vi "TCP Chat Window Launcher.vi"() -> ()   [LabVIEW 2020]
uses:
  <vilib>/NI/Actors/Network Endpoint Actors/Protocols/TCP Strategy/TCP Stream Initiator/TCP Stream Initiator.lvclass
  <vilib>/NI/Actors/Network Endpoint Actors/Protocols/TCP Strategy/TCP Stream Listener/TCP Stream Listener.lvclass
  <vilib>/NI/Actors/Network Endpoint Actors/Protocols/TCP Strategy/TCP Stream/TCP Stream.lvclass
  Chat Window/Chat Window.lvclass
  <vilib>/ActorFramework/Actor/Actor.lvclass
  C:/Program Files (x86)/National Instruments/LabVIEW 2020/vi.lib/ActorFramework/Actor/Actor.lvclass
  G:/Utilisateurs/hugofroylan.aragon/Documents/LabVIEW-Projects/Nested Endpoint Actors/Chat Window/Chat Window/Chat Window.lvclass
  C:/Program Files (x86)/National Instruments/LabVIEW 2020/vi.lib/NI/Actors/Network Endpoint Actors/Nested Endpoint Caller/Nested Endpoint Caller/Nested Endpoint Caller.lvclass
  Nested Endpoint Actors/Serializer/Serializable Flattener/Serializable Flattener.lvclass
  G:/Utilisateurs/hugofroylan.aragon/Documents/Nested Endpoint Actors Optimized/Abstract Classes/Message Flattener/Message Flattener.lvclass
  G:/Utilisateurs/hugofroylan.aragon/Documents/LabVIEW-Projects/Nested Endpoint Actors Optimized/Serializer/Serializable Flattener/Serializable Flattener.lvclass
  C:/Program Files (x86)/National Instruments/LabVIEW 2020/vi.lib/NI/Actors/Network Endpoint Actors/Protocols/TCP Strategy/TCP Stream/TCP Stream.lvclass
  G:/Utilisateurs/hugofroylan.aragon/Documents/Nested Endpoint Actors Optimized/Abstract Classes/Message Stream/Message Stream.lvclass
  C:/Program Files (x86)/National Instruments/LabVIEW 2020/vi.lib/NI/Actors/Network Endpoint Actors/Protocols/TCP Strategy/TCP Stream Listener/TCP Stream Listener.lvclass
  C:/Program Files (x86)/National Instruments/LabVIEW 2020/vi.lib/NI/Actors/Network Endpoint Actors/Protocols/TCP Strategy/TCP Stream Initiator/TCP Stream Initiator.lvclass
panel:
  out "error out":errorcluster
  in  "local port":u16=2001
  in  "Remote Port":u16=2001
  in  "Remote Address":string="127.0.0.1"
  # "This VI launches two instances of a chat window actor.  The two chat windows launch nested endpoints, which connect via a TCP/IP message stream.\n\n1.  (Optional)  Specify the IP address for this machine, and the IP ports for the two enpoints.\n2.  Run this VI.\n3.  Stop the application by closing either chat window.\n\nAF_Debug_Trace is set to TRUE in this project, so you can follow the action with the Desktop Execution Trace Toolkit."
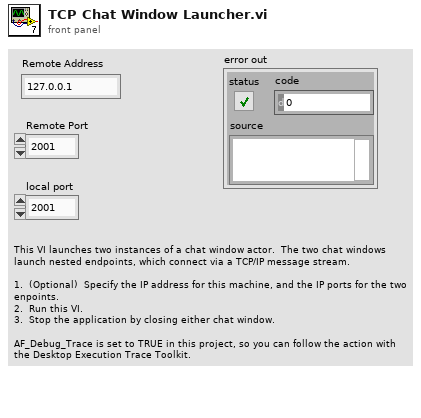
[diagram p1: front panel]
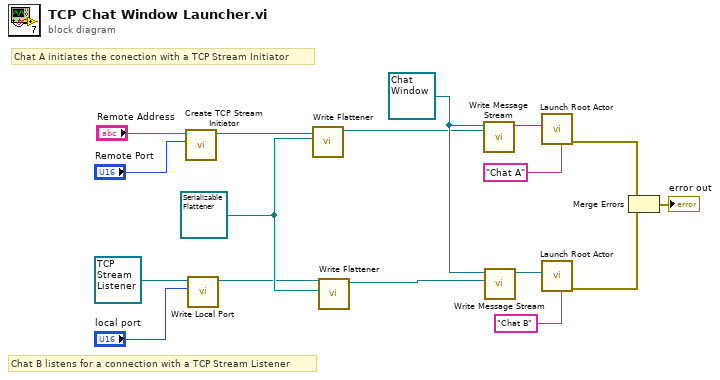
[diagram p0: block diagram]
diagram:
  w5 = refnum<class "Serializable Flattener.lvclass"> refnum ("Serializable Flattener Optimized.lvclass")
  w13 = refnum<class "Chat Window.lvclass"> refnum ("Chat Window in")
  # "Chat B listens for a connection with a TCP Stream Listener"
  # "Chat A initiates the conection with a TCP Stream Initiator"
  n1 = call <vilib>:"Create TCP Stream Initiator.vi"("Remote Port"="Remote Port", "Remote Address"="Remote Address") -> ("TCP Stream Initiator"=w3:refnum<class "TCP Stream Initiator.lvclass">)  [unwired: 9 in]
  n2 = call <vilib>:"Write Local Port.vi"("local port"="local port", "TCP Stream in"=refnum<class "TCP Stream Listener.lvclass"> refnum ("TCP Stream Listener.lvclass")) -> ("TCP Stream out"=w1:refnum<class "TCP Stream Listener.lvclass">)  [unwired: 9 in]
  n3 = call-dynamic "Write Flattener.vi"("Flattener"=w5, "TCP Stream in"=w3) -> ("TCP Stream out"=w2:refnum<class "TCP Stream Initiator.lvclass">)  [unwired: 9 in]
  n4 = call-dynamic "Write Flattener.vi"("Flattener"=w5, "TCP Stream in"=w1) -> ("TCP Stream out"=w4:refnum<class "TCP Stream Listener.lvclass">)  [unwired: 9 in]
  n5 = call "Write Message Stream.vi"("Message Stream"=w2, "Chat Window in"=w13) -> ("Chat Window out"=w12:refnum<class "Chat Window.lvclass">)  [unwired: 9 in]
  n6 = call "Write Message Stream.vi"("Message Stream"=w4, "Chat Window in"=w13) -> ("Chat Window out"=w6:refnum<class "Chat Window.lvclass">)  [unwired: 9 in]
  n7 = call <vilib>:"Launch Root Actor.vi"("Debug Alias"="Chat A", "Actor"=w12) -> ("error out"=w9:errorcluster)  [unwired: 8 in, 1 out]
  n8 = call <vilib>:"Launch Root Actor.vi"("Debug Alias"="Chat B", "Actor"=w6) -> ("error out"=w8:errorcluster)  [unwired: 8 in, 1 out]
  n9 = Merge Errors(w9, w8) -> (→"error out":errorcluster)
